vi "FM_Receiver.vi"() -> ()   [LabVIEW 2019]
uses:
  <instrlib>/niUSRP/niUSRP Fetch Rx Data (CDB WDT).vi
panel:
  in  "stop":bool
  out "Output Waveform":dynamicdata(graph)
  in  "active antenna":string
  in  "gain":dbl format="%#_6f"
  in  "carrier frequency":dbl=100000.0 format="%#_6p"
  in  "IQ rate":dbl=100000.0 format="%#_6p"
  in  "device names":refnum<k15>
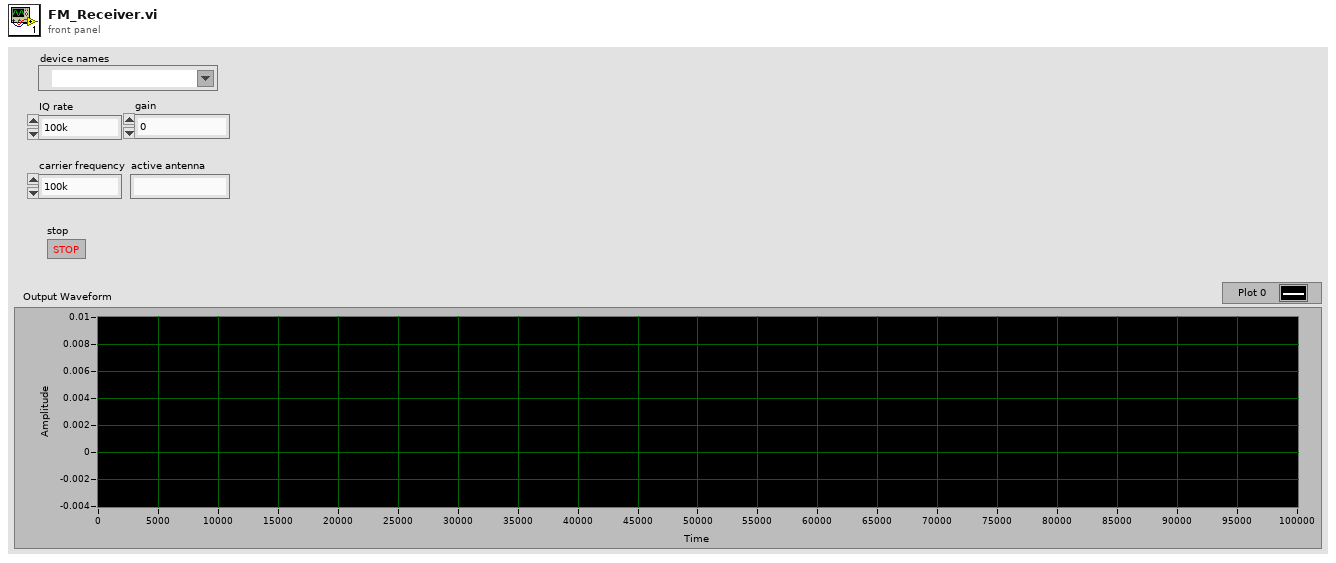
[diagram p1: front panel]
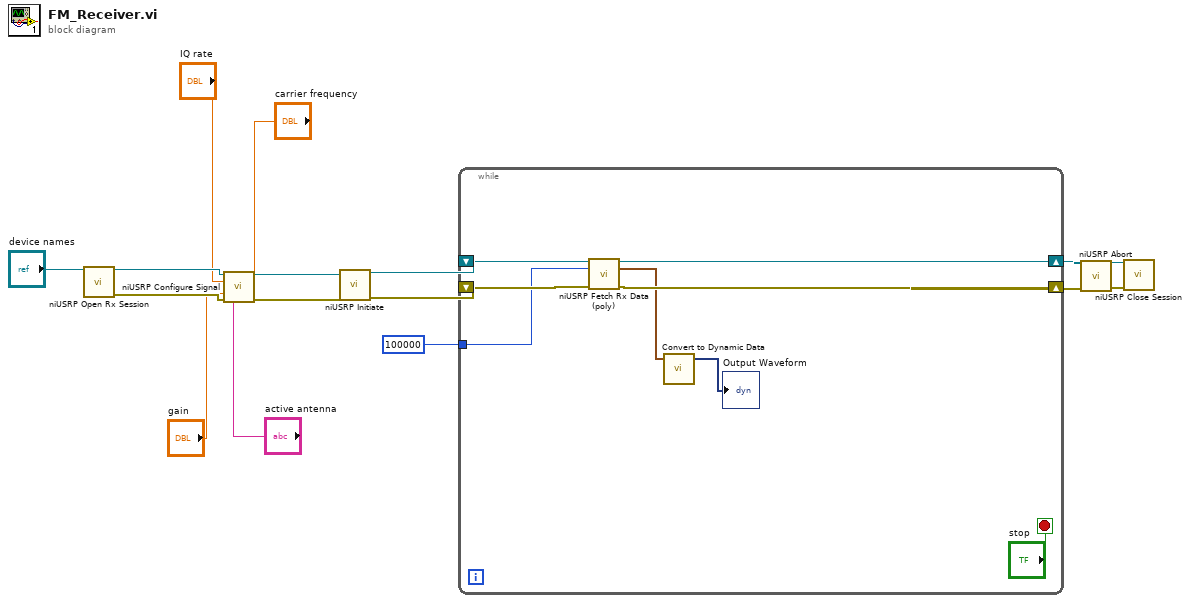
[diagram p0: block diagram]
diagram:
  n1 = call <instrlib>:"niUSRP Open Rx Session.vi"("device names"="device names") -> ("session handle out"=w16:refnum<k15>, "error out"=w12:errorcluster)  [unwired: 13 in]
  n2 = call <instrlib>:"niUSRP Configure Signal.vi"("session handle"=w16, "IQ rate"="IQ rate", "carrier frequency"="carrier frequency", "gain"="gain", "error in (no error)"=w12, "active antenna"="active antenna") -> ("session handle out"=w15:refnum<k15>, "error out"=w11:errorcluster)  [unwired: 5 in, 3 out]
  n3 = call <instrlib>:"niUSRP Initiate.vi"("session handle"=w15, "error in (no error)"=w11) -> ("session handle out"=w14:refnum<k15>, "error out"=w10:errorcluster)  [unwired: 12 in]
  n4 = while {
    shift-right: [w21] -> w2
    shift-left: w14 -> [w24]
    shift-right: [w22] -> w9
    shift-left: w10 -> [w23]
    tunnel: i64 100000 ("number of samples") -> [w20]
    stop <- "stop" stop-if-true
    n5 = call-poly <instrlib>:"niUSRP Fetch Rx Data (poly).vi"("session handle"=w24, "number of samples"=w20, "error in (no error)"=w23) -> ("session handle out"=w21:refnum<k15>, "data"=w17:waveform(cdb), "error out"=w22:errorcluster)  [unwired: 9 in, 1 out]
    n6 = call "Convert to Dynamic Data"("Array"=w17) -> ("Dynamic Data Type"=→"Output Waveform":dynamicdata)  [unwired: 3 in]
  }
  n7 = call <instrlib>:"niUSRP Abort.vi"("session handle"=w2, "error in (no error)"=w9) -> ("session handle out"=w13:refnum<k15>, "error out"=w8:errorcluster)  [unwired: 12 in]
  n8 = call <instrlib>:"niUSRP Close Session.vi"("session handle"=w13, "error in (no error)"=w8) -> ()  [unwired: 13 in, 1 out]
